vi "Constructor.vi"(5 "TimeZoneInfoId":string, 6 "MeasureExecutionStatus":T1=enum."NOT_COMPLETED", 7 "MeasureTime":timestamp, 8 "error in":errorcluster, 10 "Value":string, 11 "Name":string) -> (0 "error out":errorcluster, 3 "StringMeasure":refnum<class "StringMeasure.lvclass">)   [LabVIEW 2021, in "ProligentXMLGenerator.lvlib" / "StringMeasure.lvclass"]
uses:
  StringMeasure.lvclass
  StringMeasure.lvclass/StringMeasure.ctl
  Measure/Measure.lvclass
  Base/MeasureKind/Value.ctl
  Base/MeasureKind/MeasureKind.lvclass
  Data.ctl
  Base/String_4000/String_4000.lvclass
  C:/Projects/proligent-xml-generator-labview/src/ProligentXMLGenerator/Measure/Measure/Measure.lvclass
  C:/Projects/proligent-xml-generator-labview/src/ProligentXMLGenerator/Measure/StringMeasure/StringMeasure.lvclass
  Base/ExecutionStatus/Value.ctl
  Base/ExecutionStatus/ExecutionStatus.lvclass
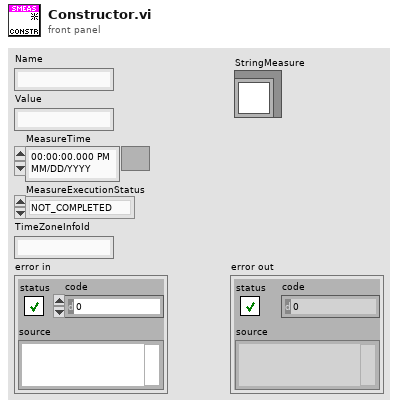
[diagram p1: front panel]
types:
  T1 = typedef "ProligentXMLGenerator.lvlib/ExecutionStatus.lvclass/Value.ctl" = enum16{"PASS", "FAIL", "NOT_COMPLETED", "ABORTED"}
  T2 = typedef "ProligentXMLGenerator.lvlib/StringMeasure.lvclass/Data.ctl" = cluster{"Value":refnum<class "String_4000.lvclass">}
  T3 = typedef "ProligentXMLGenerator.lvlib/MeasureKind.lvclass/Value.ctl" = enum16{"REAL", "BOOL", "INTEGER", "STRING", "DATETIME"}
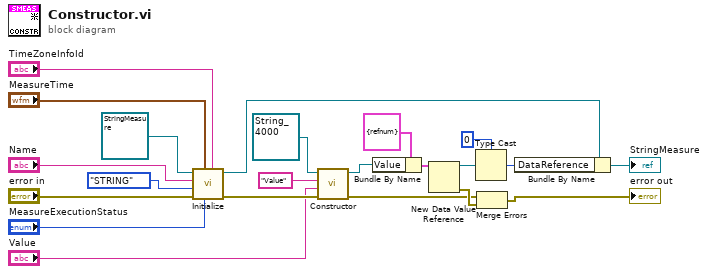
[diagram p0: block diagram]
diagram:
  n1 = call "Initialize.vi"("TimeZoneInfoId"="TimeZoneInfoId", "MeasureExecutionStatus"="MeasureExecutionStatus", "MeasureTime"="MeasureTime", "error in"="error in", "Type"=Value."STRING", "Name"="Name", "Measure in"=refnum<class "StringMeasure.lvclass"> refnum ("ProligentResultProcessor:StringMeasure")) -> ("error out"=w4:errorcluster, "Measure out"=w17:refnum<class "StringMeasure.lvclass">)  [unwired: 3 in]
  n2 = call-dynamic "Constructor.vi"("error in"=w4, "Value"="Value", "Name"="Value", "String in"=refnum<class "String_4000.lvclass"> refnum ("ProligentResultProcessor:String_4000")) -> ("error out"=w3:errorcluster, "String out"=w5:refnum<class "String_4000.lvclass">)  [unwired: 6 in]
  n3 = Bundle By Name(cluster=T2 {"Value"=refnum} ("Data"), "Value"=w5) -> (w9:T2)
  n4 = New Data Value Reference(data value=w9) -> (data value reference=w18:refnum<data-value>, error out=w21:errorcluster)  [unwired: 1 in]
  n5 = Type Cast(type=u64 0, x=w18) -> (*(type *) &x=w20:u64)
  n6 = Merge Errors(w3, w21) -> (→"error out":errorcluster)
  n7 = Bundle By Name(cluster=w17, "DataReference"=w20) -> (→"StringMeasure":refnum<class "StringMeasure.lvclass">)
